vi "doAction.vi"(8 "error in (no error)":errorcluster, 10 "ContextData":refnum<class "ContextData.lvclass">, 11 "Run in":refnum<class "Last.lvclass">) -> (0 "error out":errorcluster, 2 "ContextData Out":refnum<class "ContextData.lvclass">, 3 "Run out":refnum<class "Last.lvclass">)   [LabVIEW 2019, in "Last.lvclass"]
uses:
  Last.lvclass
  ContextData/ContextData.lvclass
  Simon_Engine/Simon_Engine.lvclass
  Messages/simonMessages/simonMessages.lvclass
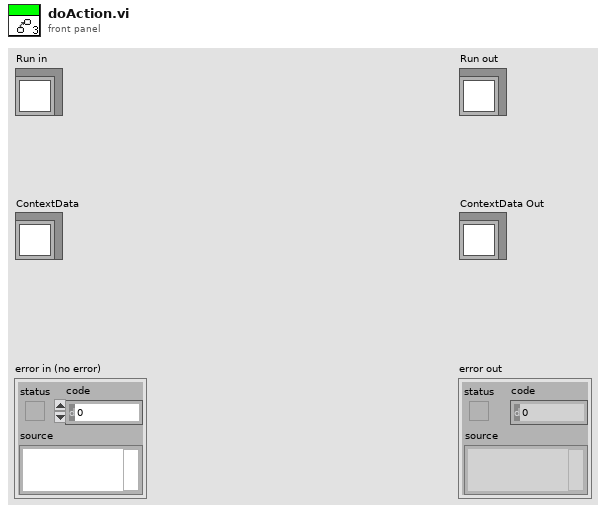
[diagram p1: front panel]
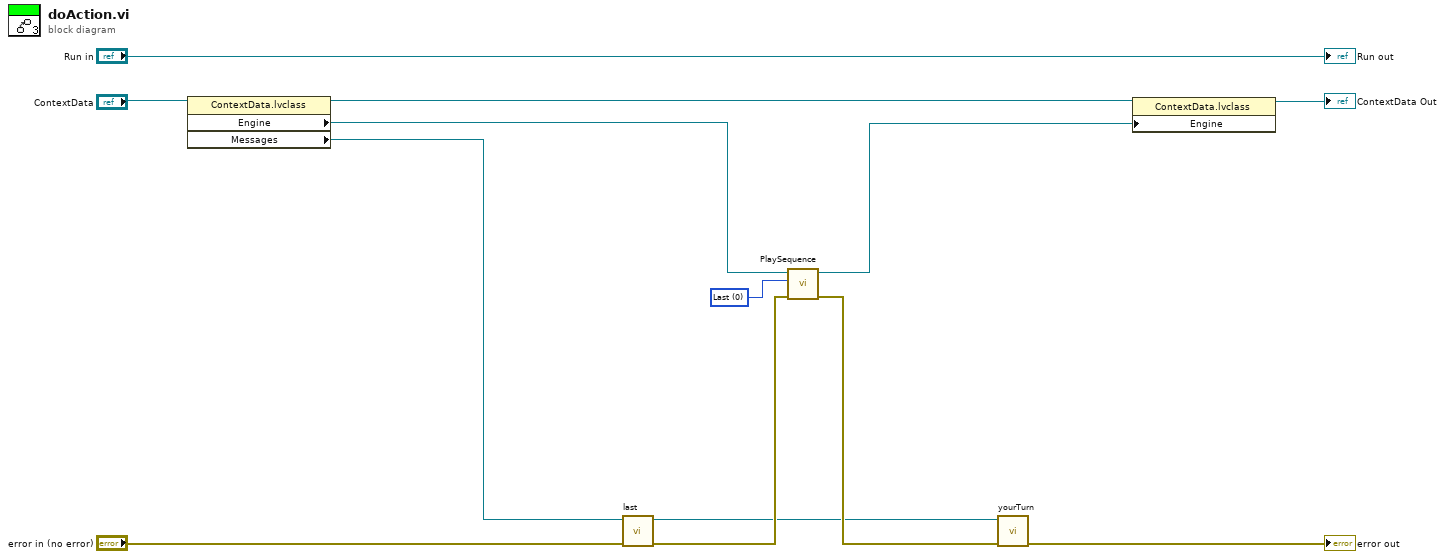
[diagram p0: block diagram]
diagram:
  w9 = u8 0 items=["Last", "Longest"] ("Sequence")
  n1 = property class="ContextData.lvclass"(reference="ContextData") -> (reference out=w6:refnum<class "ContextData.lvclass">, "Engine"=w4:refnum<class "Simon_Engine.lvclass">, "Messages"=w3:refnum<class "simonMessages.lvclass">)  [unwired: 1 in, 1 out]
  n2 = call "last.vi"("error in (no error)"="error in (no error)", "simonMessages in"=w3) -> ("error out"=w8:errorcluster, "simonMessages out"=w7:refnum<class "simonMessages.lvclass">)  [unwired: 8 in]
  n3 = call-dynamic "PlaySequence.vi"("error in (no error)"=w8, "Sequence"=w9, "Simon_Engine in"=w4) -> ("error out"=w10:errorcluster, "Simon_Engine out"=w11:refnum<class "Simon_Engine.lvclass">)  [unwired: 7 in]
  n4 = call "yourTurn.vi"("error in (no error)"=w10, "simonMessages in"=w7) -> ("error out"=→"error out":errorcluster)  [unwired: 8 in, 1 out]
  n5 = property class="ContextData.lvclass"(reference=w6, "Engine"=w11) -> (reference out=→"ContextData Out":refnum<class "ContextData.lvclass">)  [unwired: 1 in, 1 out]
  "Run out" <- "Run in"
